vi "Test Settings Editor API.vi"() -> ()   [LabVIEW 2020]
doc: "Settings Editor API Tester.\n_____\nBased on DQMH Project Template 6.0.0.91."
uses:
  DAQmx Trigger Settings--cluster.ctl
  Control 1.ctl
  DAQmx Timing--cluster.ctl
  DAQmx Config--cluster.ctl
  Settings Editor.lvlib
panel:
  in  "DAQmx Settings":T1(tab)
  out "Hardware \nConfig Cluster":T2=[{"Physical channels"="Dev1/ai0", "Channel Name"="pd", "Unit"=0, "Min Voltage"=-1.0, "Max Voltage"=1.0}] {"Unit" items=["Volts", "From Custom Scale"]}
  out "DAQmx \nTiming Settings":T3={"rate"=1000.0, "source"="OnboardClock", "sample mode"=10178, "samples per channel"=1000} {"sample mode" items=["Finite Samples"=10178, "Continuous Samples"=10123, "Hardware Timed Single Point"=12522]; "rate" format="%0.2f"}
  out "Trigger Settings":T4={"Trigger Type"=enum."No Trigger", "Digital Start"={"Source"="", "Digital Start Trigger Edge"=10280}, "Digital Pause"={"Source"="", "Digital Pause Trigger Pause When"=10192}, "Digital Reference"={"Source"="", "Digital Start Trigger Edge"=10280, "Digital Reference Pretrigger Samples"=0}, "Analog Start"={"Source"="", "Analog Slope"=10280, "Analog Start Trigger Hysteresis"=0.0, "Analog Start Trigger Level"=0.0}, "Analog Pause"={"Source"="", "Analog Start Trigger Level"=0.0, "Analog Pause Trigger Pause When"=10093}, "Analog Reference"={"Source"="", "Slope"=10280, "Pretrigger Samples"=0, "Level"=0.0}, "Time Start"={"Select Time\nManually"=FALSE, "When"=timestamp(0 s since 1904-01-01)}} {"Time Start"."When" format="%<%x %.3X>T"; "Analog Reference"."Level" format="%0.2f"; "Analog Reference"."Slope" items=["Rising"=10280, "Falling"=10171]; "Analog Pause"."Analog Pause Trigger Pause When" items=["Above Level"=10093, "Below Level"=10107]; "Analog Pause"."Analog Start Trigger Level" format="%0.2f"; "Analog Start"."Analog Start Trigger Level" format="%0.2f"; "Analog Start"."Analog Start Trigger Hysteresis" format="%.2f"; "Analog Start"."Analog Slope" items=["Rising"=10280, "Falling"=10171]; "Digital Reference"."Digital Start Trigger Edge" items=["Rising"=10280, "Falling"=10171]; "Digital Pause"."Digital Pause Trigger Pause When" items=["High"=10192, "Low"=10214]; "Digital Start"."Digital Start Trigger Edge" items=["Rising"=10280, "Falling"=10171]}
  out "Calibration Array":cluster{"Slope":dbl, "Intercept":dbl}[](array[cluster])=[{"Slope"=1.0, "Intercept"=0.0}]
  out "error out":errorcluster
  in  "Update Settings":bool
  out "Log File Base Path":path
  in  "Show Block Diagram":bool
  in  "Stop Module":bool
  in  "Start Module":bool
  in  "Hide Module Panel":bool
  in  "Show Module Panel":bool
  out "Status":string
  out "Module Running?":bool
  # "This VI tests the API for the Module."
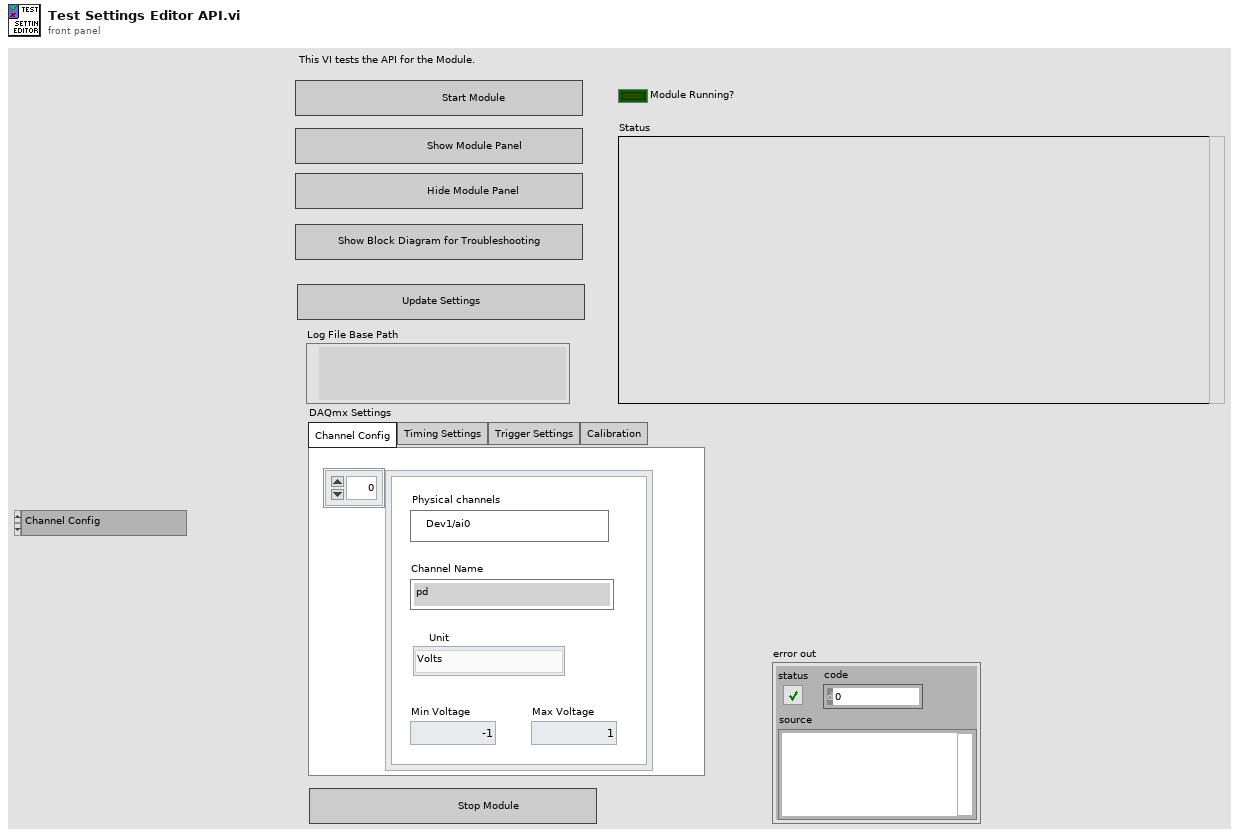
[diagram p1: front panel]
types:
  T1 = enum32{"Channel Config", "Timing Settings", "Trigger Settings", "Calibration"}
  T2 = typedef "Settings Editor.lvlib/DAQmx Config--cluster.ctl" = cluster{"Physical channels":tag, "Channel Name":string, "Unit":i32, "Min Voltage":dbl, "Max Voltage":dbl}[]
  T3 = typedef "Settings Editor.lvlib/DAQmx Timing--cluster.ctl" = cluster{"rate":dbl, "source":tag, "sample mode":i32, "samples per channel":i32}
  T4 = typedef "Settings Editor.lvlib/DAQmx Trigger Settings--cluster.ctl" = cluster{"Trigger Type":enum32{"No Trigger", "Digital Start", "Digital Pause", "Digital Reference", "Analog Start", "Analog Pause", "Analog Reference", "Time Start"}, "Digital Start":cluster{"Source":tag, "Digital Start Trigger Edge":i32}, "Digital Pause":cluster{"Source":tag, "Digital Pause Trigger Pause When":i32}, "Digital Reference":cluster{"Source":tag, "Digital Start Trigger Edge":i32, "Digital Reference Pretrigger Samples":u32}, "Analog Start":cluster{"Source":string, "Analog Slope":i32, "Analog Start Trigger Hysteresis":dbl, "Analog Start Trigger Level":dbl}, "Analog Pause":cluster{"Source":string, "Analog Start Trigger Level":dbl, "Analog Pause Trigger Pause When":i32}, "Analog Reference":T5, "Time Start":cluster{"Select Time\nManually":bool, "When":timestamp}}
  T5 = typedef "Control 1.ctl" = cluster{"Source":string, "Slope":i32, "Pretrigger Samples":u32, "Level":dbl}
  T6 = typedef "Settings Editor.lvlib/Broadcast Events--cluster.ctl" = cluster{"Module Did Init":refnum<user-event>, "Status Updated":refnum<user-event>, "Error Reported":refnum<user-event>, "Module Did Stop":refnum<user-event>, "Update Module Execution Status":refnum<user-event>, "Application Settings Updated":refnum<user-event>}
  T7 = typedef "Settings Editor.lvlib/Update Application Settings (Reply Payload)--cluster.ctl" = cluster{"Settings":T8, "Update Settings_error":errorcluster}
  T8 = typedef "Settings Editor.lvlib/Settings--cluster.ctl" = cluster{"Calibration Array":cluster{"Slope":dbl, "Offset":dbl}[], "Hardware Config Cluster":T2, "Trigger Settings":T4, "Log File Base Path":path, "DAQmx Timing Settings":T3}
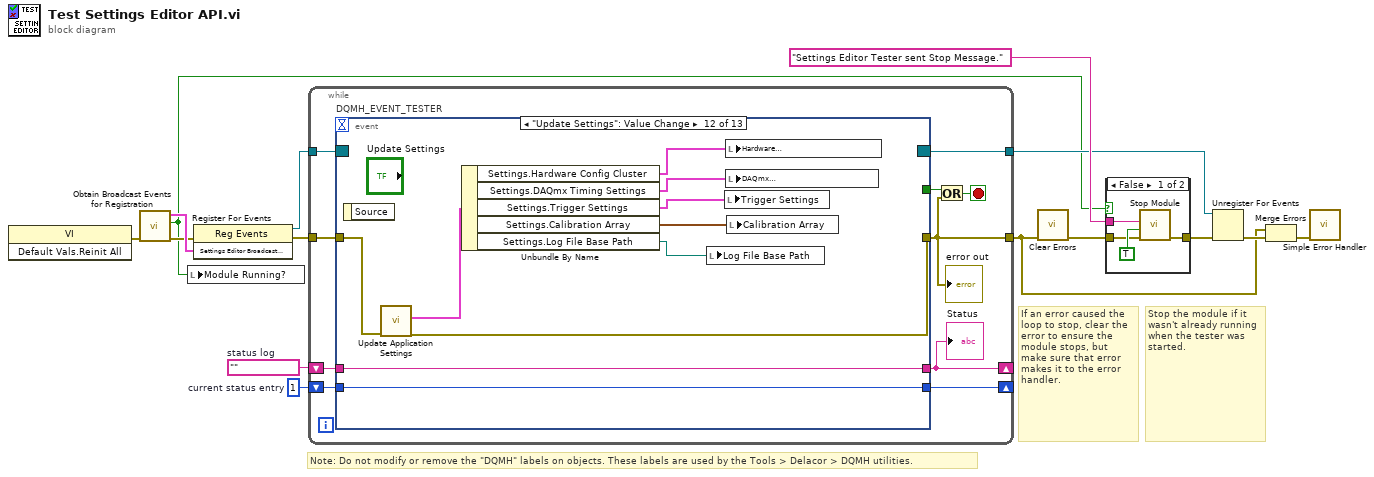
[diagram p0: block diagram]
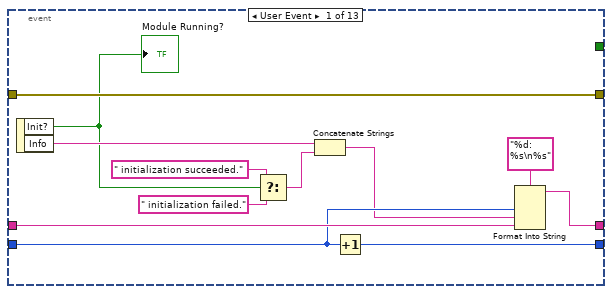
[diagram p3: hidden frame]
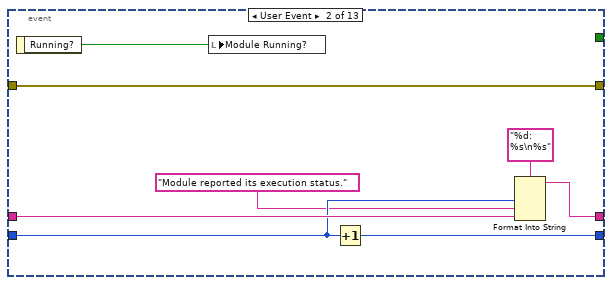
[diagram p4: hidden frame]
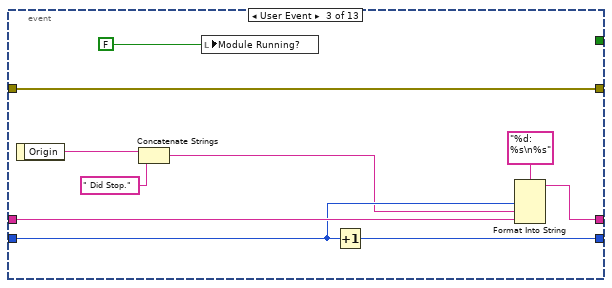
[diagram p5: hidden frame]
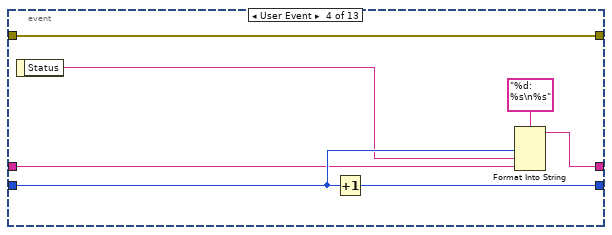
[diagram p6: hidden frame]
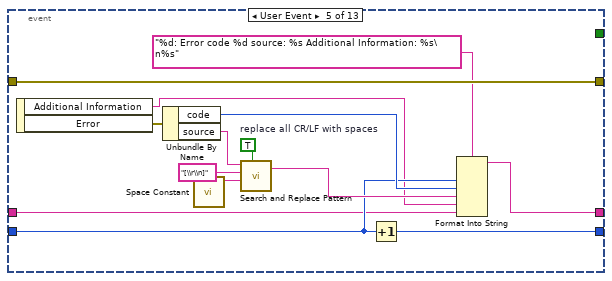
[diagram p7: hidden frame]
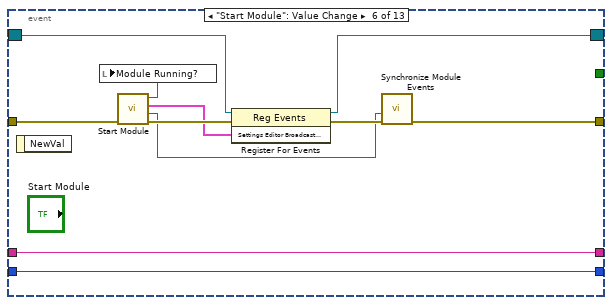
[diagram p8: hidden frame]
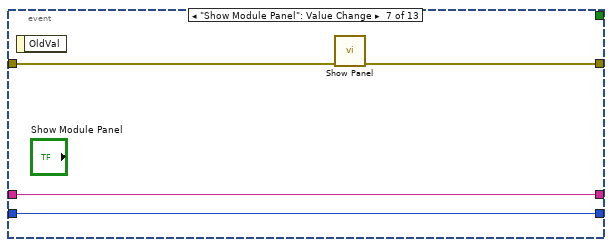
[diagram p9: hidden frame]
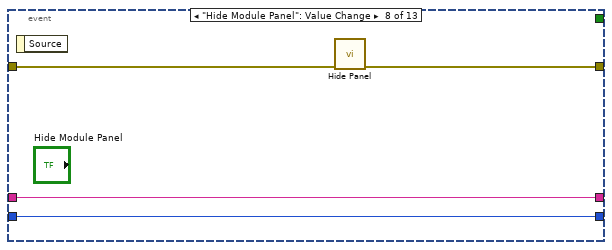
[diagram p10: hidden frame]
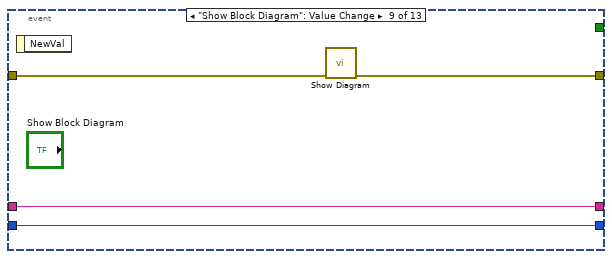
[diagram p11: hidden frame]
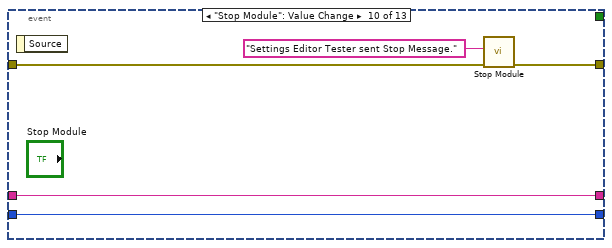
[diagram p12: hidden frame]
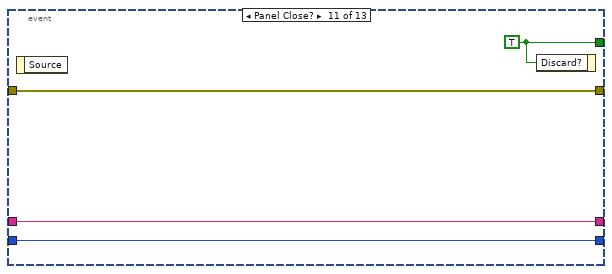
[diagram p13: hidden frame]
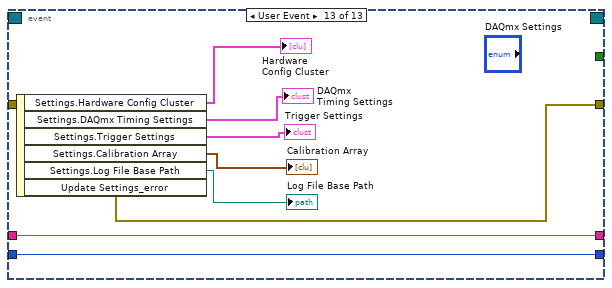
[diagram p14: hidden frame]
diagram:
  w11 = 1  # current status entry
  w12 = ""  # status log
  # "Stop the module if it wasn't already running when the tester was started."
  # "If an error caused the loop to stop, clear the error to ensure the module stops, but make sure that error makes it to the error handler."
  # "Note: Do not modify or remove the \"DQMH\" labels on objects. These labels are used by the Tools > Delacor > DQMH utilities."
  n1 = invoke class="VI" method="Default Vals.Reinit All"() -> (error out=w3:errorcluster)  [unwired: 3 in, 2 out]
  n2 = call "Obtain Broadcast Events for Registration.vi"("error in (no error)"=w3) -> ("error out"=w2:errorcluster, "Already running?"=w1:bool, "Settings Editor Broadcast Events"=w9:T6)  [unwired: 8 in]
  n3 = local write "Module Running?"(w1) -> ()
  n4 = register-events(error in=w2, w9) -> (reference out=w8:refnum<event-registration>, error out=w10:errorcluster)  [unwired: 1 in]
  n5 = while {
    tunnel: w8 -> [w25]
    tunnel: [w16] -> w4
    shift-right: [w20] -> _
    shift-left: w12 -> [w22]
    shift-right: [w21] -> _
    shift-left: w11 -> [w23]
    tunnel: w10 -> [w18]
    tunnel: [w17] -> w7
    stop <- w19 stop-if-true
    n6 = event "DQMH_EVENT_TESTER" shown="[11] \"Update Settings\": Value Change" {
      selector: w25 -> [_ _ _ _ _ w81 _ _ _ _ _ _ _]
      dyn-events: [_ _ _ _ _ w80 _ _ _ _ _ _ _] -> w17
      timeout: _ -> [_ _ _ _ _ _ _ _ _ _ _ _ _]
      tunnel: [_ _ _ _ _ _ _ _ _ _ w108 _ _] -> w24
      tunnel: [w37 w39 w46 w56 w76 w79 w91 w95 w96 w102 w105 w115 w124] -> w16
      tunnel: w23 -> [w34 w43 w53 w59 w66 w84 w89 w93 w97 w103 w106 w116 w125]
      tunnel: w22 -> [w35 w44 w54 w58 w64 w85 w90 w94 w98 w104 w107 w117 w126]
      tunnel: [w32 w41 w51 w60 w67 w85 w90 w94 w98 w104 w107 w117 w126] -> w20
      tunnel: [w33 w42 w52 w62 w65 w84 w89 w93 w97 w103 w106 w116 w125] -> w21
      tunnel: w18 -> [w37 w39 w46 w56 w76 w78 w88 w92 w99 w100 w105 w118 _]
      event User Event {
        n7 = event-data() -> ("Init?"=w29:bool, "Info"=w31:string)  [unwired: 1 in]
        "Module Running?" <- w29
        n8 = Select(t=" initialization succeeded.", s=w29, f=" initialization failed.") -> (s? t:f=w26:string)
        n9 = Concatenate Strings(w31, w26) -> (w30:string)
        n10 = Increment(x=w34) -> (x+1=w33:i32)
        n11 = Format Into String(format string="%d: %s\n%s", w34, w30, w35) -> (resulting string=w32:string)  [unwired: 2 in, 1 out]
      }
      event User Event {
        n12 = event-data() -> ("Running?"=w38:bool)  [unwired: 1 in]
        n13 = local write "Module Running?"(w38) -> ()
        n14 = Increment(x=w43) -> (x+1=w42:i32)
        n15 = Format Into String(format string="%d: %s\n%s", w43, "Module reported its execution status.", w44) -> (resulting string=w41:string)  [unwired: 2 in, 1 out]
      }
      event User Event {
        n16 = event-data() -> ("Origin"=w50:string)  [unwired: 1 in]
        n17 = Concatenate Strings(w50, " Did Stop.") -> (w49:string)
        n18 = local write "Module Running?"(FALSE ("Module Did Init?")) -> ()
        n19 = Increment(x=w53) -> (x+1=w52:i32)
        n20 = Format Into String(format string="%d: %s\n%s", w53, w49, w54) -> (resulting string=w51:string)  [unwired: 2 in, 1 out]
      }
      event User Event {
        n21 = event-data() -> ("Status"=w57:string)  [unwired: 1 in]
        n22 = Increment(x=w59) -> (x+1=w62:i32)
        n23 = Format Into String(format string="%d: %s\n%s", w59, w57, w58) -> (resulting string=w60:string)  [unwired: 2 in, 1 out]
      }
      event User Event {
        w72 = TRUE  # replace all CR/LF with spaces
        n24 = event-data() -> ("Additional Information"=w63:string, "Error"=w68:errorcluster)  [unwired: 1 in]
        n25 = Unbundle By Name(w68) -> ("code"=w69:i32, "source"=w70:string)
        n26 = call <vilib>:"Space Constant.vi"() -> ("String"=w73:string)
        n27 = call <vilib>:"Search and Replace Pattern.vi"("string"=w70, "regular expression (\"\")"="[\\r\\n]" ("regular expression (\"\")"), "replace string (\"\")"=w73, "replace all? (F)"=w72) -> ("result string"=w71:string)  [unwired: 1 in, 1 out]
        n28 = Increment(x=w66) -> (x+1=w65:i32)
        n29 = Format Into String(format string="%d: Error code %d source: %s Additional Information: %s\n%s", w66, w69, w71, w63, w64) -> (resulting string=w67:string)  [unwired: 2 in, 1 out]
      }
      event "Start Module": Value Change {
        n30 = event-data() -> ()  [unwired: 1 in, 1 out]
        n31 = call "Start Module.vi"("error in (no error)"=w78) -> ("error out"=w86:errorcluster, "Wait for Event Sync?"=w83:bool, "Settings Editor Broadcast Events"=w82:T6, "Module Was Already Running?"=w77:bool)  [unwired: 7 in]
        n32 = local write "Module Running?"(w77) -> ()
        n33 = register-events(reference=w81, error in=w86, w82) -> (reference out=w80:refnum<event-registration>, error out=w87:errorcluster)
        n34 = call "Synchronize Module Events.vi"("error in (no error)"=w87, "Wait for Event Sync?"=w83) -> ("error out"=w79:errorcluster)  [unwired: 9 in]
      }
      event "Show Module Panel": Value Change {
        n35 = event-data() -> ()  [unwired: 1 in, 1 out]
        n36 = call "Show Panel.vi"("error in (no error)"=w88) -> ("error out"=w91:errorcluster)  [unwired: 10 in]
      }
      event "Hide Module Panel": Value Change {
        n37 = event-data() -> ()  [unwired: 1 in, 1 out]
        n38 = call "Hide Panel.vi"("error in (no error)"=w92) -> ("error out"=w95:errorcluster)  [unwired: 10 in]
      }
      event "Show Block Diagram": Value Change {
        n39 = event-data() -> ()  [unwired: 1 in, 1 out]
        n40 = call "Show Diagram.vi"("error in (no error)"=w99) -> ("error out"=w96:errorcluster)  [unwired: 10 in]
      }
      event "Stop Module": Value Change {
        n41 = event-data() -> ()  [unwired: 1 in, 1 out]
        n42 = call "Stop Module.vi"("error in (no error)"=w100, "Origin"="Settings Editor Tester sent Stop Message.") -> ("error out"=w102:errorcluster)  [unwired: 9 in]
      }
      event Panel Close? {
        w108 = TRUE ("Discard?")
        n43 = event-data() -> ()  [unwired: 1 in, 1 out]
        n44 = event-data("Discard?"=w108) -> ()  [unwired: 1 in, 1 out]
      }
      event "Update Settings": Value Change {
        n45 = event-data() -> ()  [unwired: 1 in, 1 out]
        n46 = call "Update Application Settings.vi"("error in (no error)"=w118) -> ("error out"=w115:errorcluster, "Reply Payload"=w114:T7)  [unwired: 8 in, 1 out]
        n47 = Unbundle By Name(w114) -> ("Settings.Hardware Config Cluster"=w109:T2, "Settings.DAQmx Timing Settings"=w110:T3, "Settings.Trigger Settings"=w111:T4, "Settings.Calibration Array"=w112:cluster{"Slope":dbl, "Offset":dbl}[], "Settings.Log File Base Path"=w113:path)
        n48 = local write "Log File Base Path"(w113) -> ()
        n49 = local write "Trigger Settings"(w111) -> ()
        n50 = local write "Hardware \nConfig Cluster"(w109) -> ()
        n51 = local write "DAQmx \nTiming Settings"(w110) -> ()
        n52 = local write "Calibration Array"(w112) -> ()
      }
      event User Event {
        n53 = event-data() -> ("Settings.Hardware Config Cluster"=→"Hardware \nConfig Cluster":T2, "Settings.DAQmx Timing Settings"=→"DAQmx \nTiming Settings":T3, "Settings.Trigger Settings"=→"Trigger Settings":T4, "Settings.Calibration Array"=→"Calibration Array":cluster{"Slope":dbl, "Offset":dbl}[], "Settings.Log File Base Path"=→"Log File Base Path":path, "Update Settings_error"=w124:errorcluster)  [unwired: 1 in]
      }
    }
    "Status" <- w20
    "error out" <- w16
    n54 = Or(x=w24, y=w16) -> (x .or. y?=w19:bool)
  }
  n55 = call <vilib>:"Clear Errors.vi"("error in (no error)"=w4) -> ("error out"=w6:errorcluster)  [unwired: 5 in, 1 out]
  n56 = case shown="False" w1 {
    tunnel: [w130 w131] -> w14
    tunnel: "Settings Editor Tester sent Stop Message." ("Origin") -> [w129 _]
    tunnel: w6 -> [w127 w131]
    frame False {
      n57 = call "Stop Module.vi"("error in (no error)"=w127, "Wait for Module to Stop? (F)"=TRUE ("Wait for Module to stop?"), "Origin"=w129) -> ("error out"=w130:errorcluster)  [unwired: 8 in]
    }
    frame True {
    }
  }
  n58 = Unregister For Events(event registration refnum=w7, error in=w14) -> (error out=w15:errorcluster)
  n59 = Merge Errors(w4, w15) -> (w5:errorcluster)
  n60 = call <vilib>:"Simple Error Handler.vi"("error in (no error)"=w5) -> ()  [unwired: 4 in, 5 out]
